vi "F3.vi"(8 "s":dbl, 9 "d":dbl, 10 "w":dbl, 11 "a":dbl) -> (2 "F3":dbl format="%#_13g")   [LabVIEW 2021]
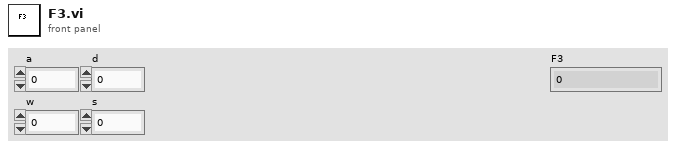
[diagram p1: front panel]
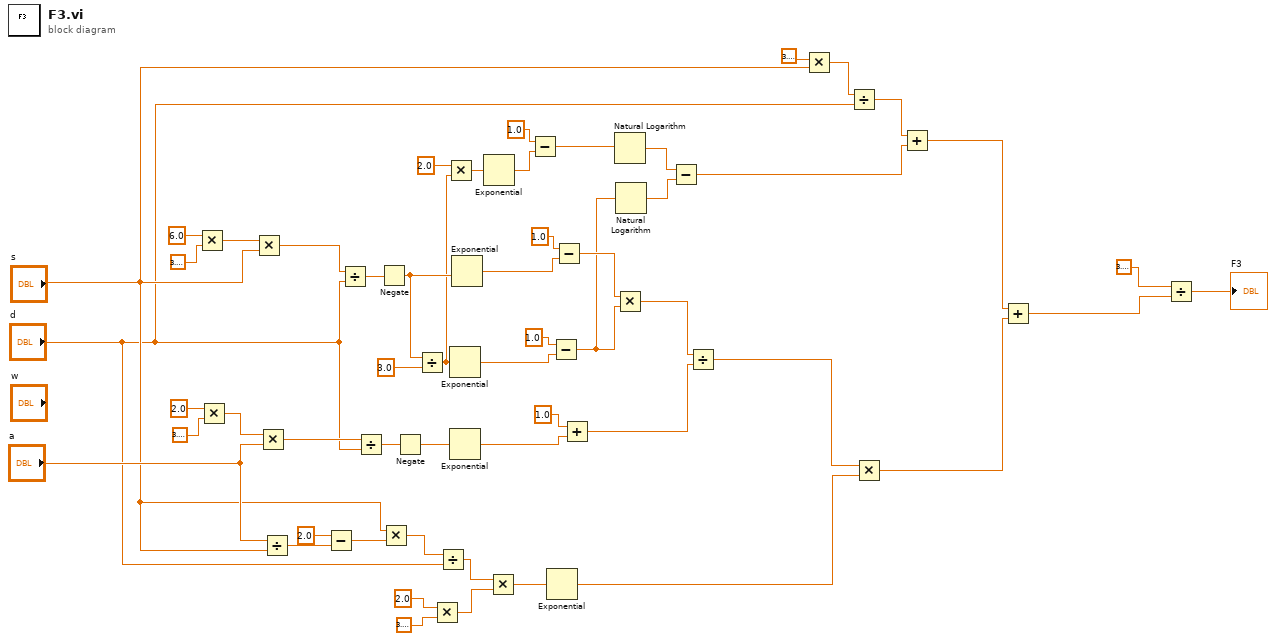
[diagram p0: block diagram]
diagram:
  n1 = Multiply(x=6.0, y=3.141592653589793) -> (x*y=w52:dbl)
  n2 = Multiply(x=2.0, y=3.141592653589793) -> (x*y=w40:dbl)
  n3 = Multiply(x=w52, y="s") -> (x*y=w51:dbl)
  n4 = Multiply(x=w40, y="a") -> (x*y=w39:dbl)
  n5 = Divide(x="a", y="s") -> (x/y=w28:dbl)
  n6 = Subtract(x=2.0, y=w28) -> (x-y=w26:dbl)
  n7 = Divide(x=w51, y="d") -> (x/y=w48:dbl)
  n8 = Divide(x=w39, y="d") -> (x/y=w38:dbl)
  n9 = Negate(x=w48) -> (-x=w43:dbl)
  n10 = Multiply(x="s", y=w26) -> (x*y=w25:dbl)
  n11 = Negate(x=w38) -> (-x=w37:dbl)
  n12 = Divide(x=w43, y=3.0) -> (x/y=w21:dbl)
  n13 = Multiply(x=2.0, y=3.141592653589793) -> (x*y=w23:dbl)
  n14 = Divide(x=w25, y="d") -> (x/y=w24:dbl)
  n15 = Multiply(x=2.0, y=w21) -> (x*y=w19:dbl)
  n16 = Exponential(1:w21) -> (0:w46:dbl)
  n17 = Exponential(1:w37) -> (0:w36:dbl)
  n18 = Exponential(1:w43) -> (0:w50:dbl)
  n19 = Exponential(1:w19) -> (0:w17:dbl)
  n20 = Multiply(x=w24, y=w23) -> (x*y=w2:dbl)
  n21 = Subtract(x=1.0, y=w17) -> (x-y=w16:dbl)
  n22 = Exponential(1:w2) -> (0:w1:dbl)
  n23 = Subtract(x=1.0, y=w46) -> (x-y=w22:dbl)
  n24 = Subtract(x=1.0, y=w50) -> (x-y=w44:dbl)
  n25 = Add(x=1.0, y=w36) -> (x+y=w33:dbl)
  n26 = Natural Logarithm(1:w16) -> (0:w14:dbl)
  n27 = Multiply(x=w44, y=w22) -> (x*y=w34:dbl)
  n28 = Natural Logarithm(1:w22) -> (0:w15:dbl)
  n29 = Subtract(x=w14, y=w15) -> (x-y=w8:dbl)
  n30 = Divide(x=w34, y=w33) -> (x/y=w32:dbl)
  n31 = Multiply(x=3.141592653589793, y="s") -> (x*y=w11:dbl)
  n32 = Divide(x=w11, y="d") -> (x/y=w9:dbl)
  n33 = Multiply(x=w32, y=w1) -> (x*y=w6:dbl)
  n34 = Add(x=w9, y=w8) -> (x+y=w7:dbl)
  n35 = Add(x=w7, y=w6) -> (x+y=w4:dbl)
  n36 = Divide(x=3.141592653589793, y=w4) -> (x/y=→"F3":dbl)
